vi "MonitorVoltaje&Frecuencia.vi"(8 "error in (no error)":errorcluster, 10 "Cluster":T1, 11 "Prueba33 in":refnum<class "Prueba33.lvclass">) -> (0 "error out":errorcluster, 3 "Prueba33 out":refnum<class "Prueba33.lvclass">)   [LabVIEW 2019, in "Prueba33.lvclass"]
uses:
  Prueba33.lvclass
  Prueba33.lvclass/Prueba33.ctl
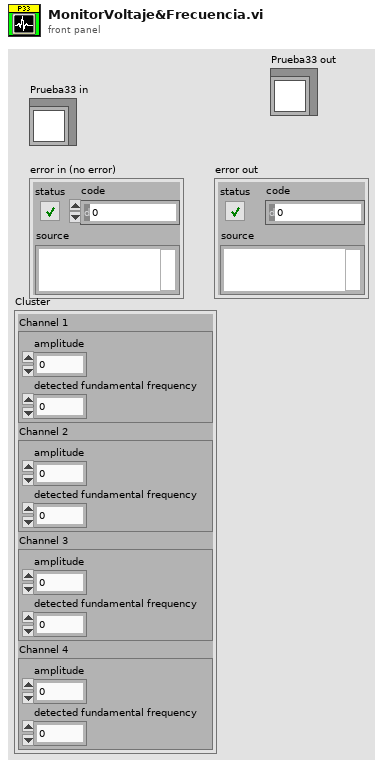
[diagram p1: front panel]
types:
  T1 = cluster{"Channel 1":cluster{"amplitude":dbl, "detected fundamental frequency":dbl}, "Channel 2":cluster{"amplitude":dbl, "detected fundamental frequency":dbl}, "Channel 3":cluster{"amplitude":dbl, "detected fundamental frequency":dbl}, "Channel 4":cluster{"amplitude":dbl, "detected fundamental frequency":dbl}}
  T2 = cluster{"ControlName":string, "ControlReference":refnum<vi>}[]
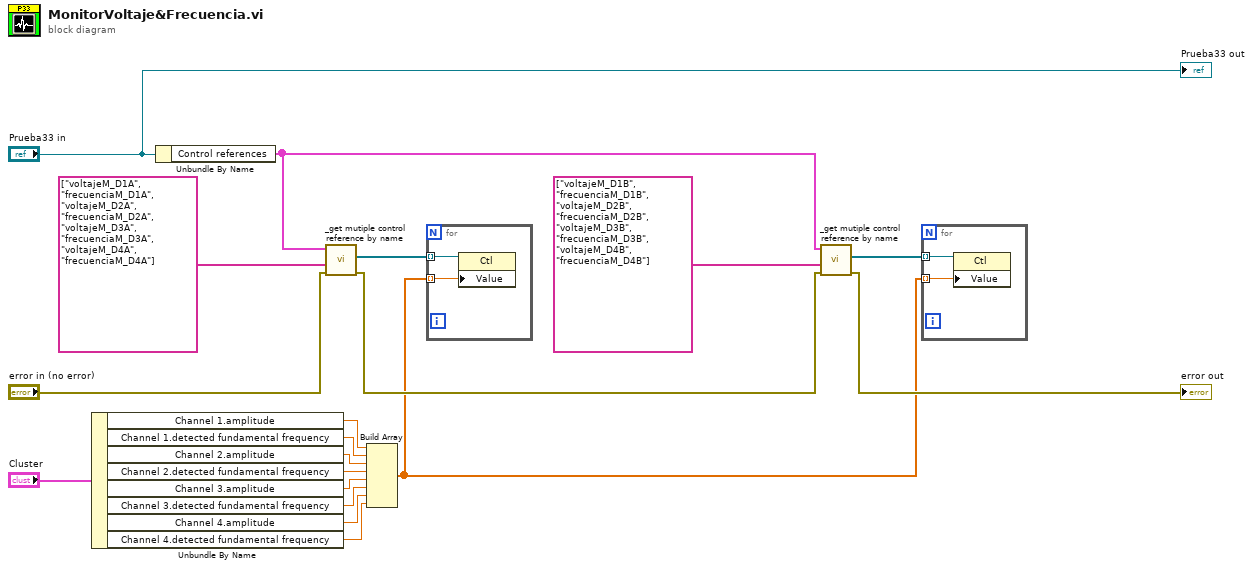
[diagram p0: block diagram]
diagram:
  n1 = Unbundle By Name("Cluster") -> ("Channel 1.amplitude"=w14:dbl, "Channel 1.detected fundamental frequency"=w13:dbl, "Channel 2.amplitude"=w12:dbl, "Channel 2.detected fundamental frequency"=w11:dbl, "Channel 3.amplitude"=w10:dbl, "Channel 3.detected fundamental frequency"=w9:dbl, "Channel 4.amplitude"=w8:dbl, "Channel 4.detected fundamental frequency"=w7:dbl)
  n2 = Unbundle By Name("Prueba33 in") -> ("Control references"=w6:T2)
  n3 = call "_get mutiple control reference by name.vi"("error in (no error)"="error in (no error)", "Control names"=string[] ["voltajeM_D1A", "frecuenciaM_D1A", "voltajeM_D2A", "frecuenciaM_D2A", "voltajeM_D3A", "frecuenciaM_D3A", "voltajeM_D4A", "frecuenciaM_D4A"], "Control references"=w6) -> ("error out"=w4:errorcluster, "References"=w16:refnum<vi>[])  [unwired: 3 in]
  n4 = Build Array(w14, w13, w12, w11, w10, w9, w8, w7) -> (w1:dbl[])
  n5 = for {
    tunnel: w16 -> [w21] mode=indexing
    tunnel: w1 -> [w20] mode=indexing
    n6 = property class="Ctl"(reference=w21, "Value"=w20) -> ()  [unwired: 1 in, 2 out]
  }
  n7 = call "_get mutiple control reference by name.vi"("error in (no error)"=w4, "Control names"=string[] ["voltajeM_D1B", "frecuenciaM_D1B", "voltajeM_D2B", "frecuenciaM_D2B", "voltajeM_D3B", "frecuenciaM_D3B", "voltajeM_D4B", "frecuenciaM_D4B"], "Control references"=w6) -> ("error out"=→"error out":errorcluster, "References"=w2:refnum<vi>[])  [unwired: 3 in]
  n8 = for {
    tunnel: w2 -> [w23] mode=indexing
    tunnel: w1 -> [w22] mode=indexing
    n9 = property class="Ctl"(reference=w23, "Value"=w22) -> ()  [unwired: 1 in, 2 out]
  }
  "Prueba33 out" <- "Prueba33 in"
